vi "Simulated data.vi"(8 "error in":errorcluster, 10 "Data format":enum16{"IDRA data", "XAM data"}(ring), 11 "run/reset":bool=TRUE) -> (0 "error out":errorcluster, 3 "Array":u8[](array[numeric]))   [LabVIEW 2015, in "Acquisition.lvlib"]
uses:
  Acquisition/Acquisition.lvlib
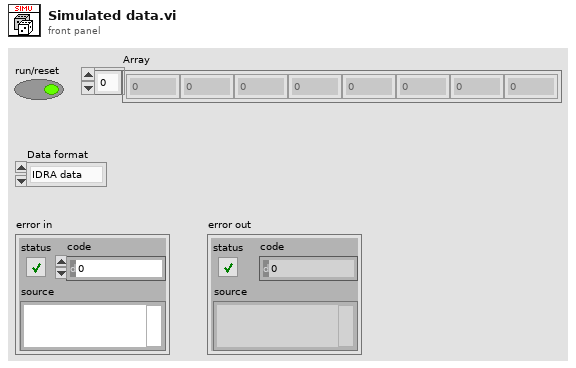
[diagram p1: front panel]
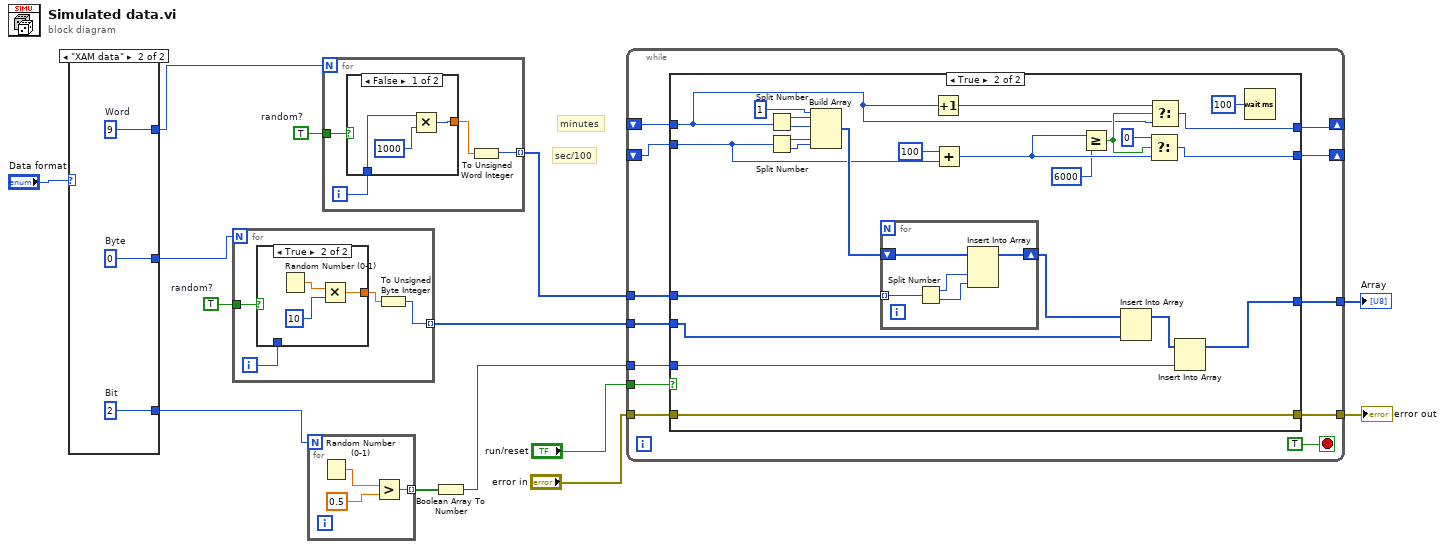
[diagram p0: block diagram]
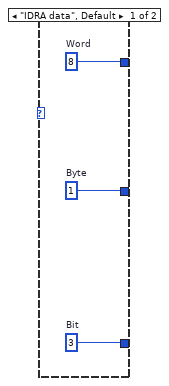
[diagram p2: hidden frame]
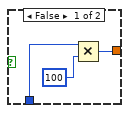
[diagram p3: hidden frame]
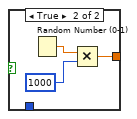
[diagram p4: hidden frame]
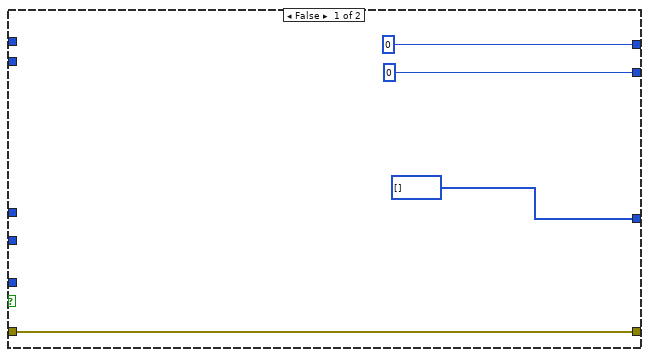
[diagram p5: hidden frame]
diagram:
  w6 = TRUE  # random?
  w9 = TRUE  # random?
  # "sec/100"
  # "minutes"
  n1 = case shown="\"XAM data\"" "Data format" {
    tunnel: [w15 w20] -> w3
    tunnel: [w16 w19] -> w2
    tunnel: [w17 w18] -> w1
    frame "IDRA data", Default {
      w15 = 3  # Bit
      w17 = 8  # Word
      w16 = 1  # Byte
    }
    frame "XAM data" {
      w20 = 2  # Bit
      w18 = 9  # Word
      w19 = 0  # Byte
    }
  }
  n2 = for {
    N: w2 -> [_]
    tunnel: [w22] -> w5 mode=indexing
    tunnel: w6 -> [w24]
    i -> [w23]
    n3 = case shown="True" w24 {
      tunnel: w23 -> [w27 _]
      tunnel: [w25 w28] -> w21
      frame False {
        n4 = Multiply(x=w27, y=100) -> (x*y=w25:i32)
      }
      frame True {
        n5 = Random Number (0-1)() -> (number: 0 to 1=w30:dbl)
        n6 = Multiply(x=w30, y=u16 10) -> (x*y=w28:dbl)
      }
    }
    n7 = To Unsigned Byte Integer(number=w21) -> (unsigned 8bit integer=w22:u8)
  }
  n8 = for {
    N: w3 -> [_]
    tunnel: [w31] -> w8 mode=indexing
    n9 = Random Number (0-1)() -> (number: 0 to 1=w33:dbl)
    n10 = Greater?(x=w33, y=0.5) -> (0:w31:bool)
  }
  n11 = for {
    N: w1 -> [_]
    tunnel: [w35] -> w10 mode=indexing
    tunnel: w9 -> [w37]
    i -> [w36]
    n12 = case shown="False" w37 {
      tunnel: w36 -> [w40 _]
      tunnel: [w38 w41] -> w34
      frame False {
        n13 = Multiply(x=w40, y=1000) -> (x*y=w38:i32)
      }
      frame True {
        n14 = Random Number (0-1)() -> (number: 0 to 1=w43:dbl)
        n15 = Multiply(x=w43, y=u16 1000) -> (x*y=w41:dbl)
      }
    }
    n16 = To Unsigned Word Integer(number=w34) -> (unsigned 16bit integer=w35:u16)
  }
  n17 = Boolean Array To Number(Boolean array=w8) -> (number=w7:u32)
  n18 = while {
    shift-right: [w52] -> _
    shift-left: _ -> [w51]
    tunnel: w10 -> [w54]
    tunnel: "run/reset" -> [w53]
    tunnel: "error in" -> [w50]
    tunnel: [w49] -> w12
    tunnel: w7 -> [w48]
    tunnel: [w47] -> w11
    shift-right: [w46] -> _
    shift-left: _ -> [w45]
    tunnel: w5 -> [w44]
    stop <- TRUE stop-if-true
    n19 = case shown="True" w53 {
      tunnel: w54 -> [_ w83]
      tunnel: [u16 0 w69] -> w52
      tunnel: w51 -> [_ w67]
      tunnel: w50 -> [w58 w77]
      tunnel: [w58 w77] -> w49
      tunnel: w48 -> [_ w63]
      tunnel: [u16[] [] w75] -> w47
      tunnel: [u16 0 w70] -> w46
      tunnel: w45 -> [_ w74]
      tunnel: w44 -> [_ w62]
      frame False {
      }
      frame True {
        n20 = Split Number(x=w67) -> (hi(x)=w82:u8, lo(x)=w81:u8)
        n21 = Split Number(x=w74) -> (hi(x)=w80:u8, lo(x)=w79:u8)
        n22 = Build Array(u8 1 ("element"), w82, w81, w80, w79) -> (w76:u8[])
        n23 = for {
          tunnel: w83 -> [w84] mode=indexing
          shift-right: [w85] -> w61
          shift-left: w76 -> [w88]
          n24 = Split Number(x=w84) -> (hi(x)=w87:u8, lo(x)=w86:u8)
          n25 = Insert Into Array(array=w88, new element #1=w87, new element #2=w86) -> (w85:u8[])  [unwired: 1 in]
        }
        n26 = Increment(x=w67) -> (x+1=w66:u16)
        n27 = Add(x=u16 100, y=w74) -> (x+y=w72:u16)
        n28 = Greater Or Equal?(x=w72, y=u16 6000 ("x")) -> (x >= y?=w68:bool)
        n29 = Insert Into Array(array=w61, new element=w62) -> (w60:u8[])  [unwired: 1 in]
        n30 = Select(t=u16 0, s=w68, f=w72) -> (s? t:f=w70:u16)
        n31 = Select(t=w66, s=w68, f=w67) -> (s? t:f=w69:u16)
        n32 = Insert Into Array(array=w60, new element=w63) -> (w75:u8[])  [unwired: 1 in]
        n33 = Wait (ms)(milliseconds to wait=u32 100) -> ()  [unwired: 1 out]
      }
    }
  }
  "error out" <- w12
  "Array" <- w11
